vi "Save File DOE Find Individual Elements.vi"(11 "Input Array":string[](array[string])=["A", "a", "a", "B", "B", "c", "c", "C", "D", "E", "F", "F", "F", "G"]) -> (3 "Individual Elements":string[](array[string]))   [LabVIEW 2016, in "File Setup.lvlib"]
uses:
  File Setup.lvlib
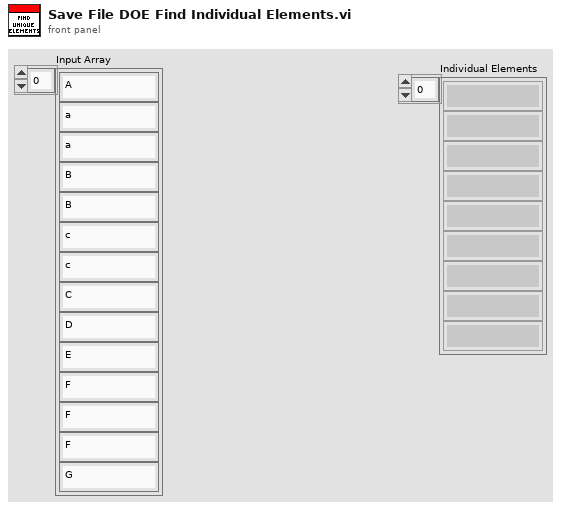
[diagram p1: front panel]
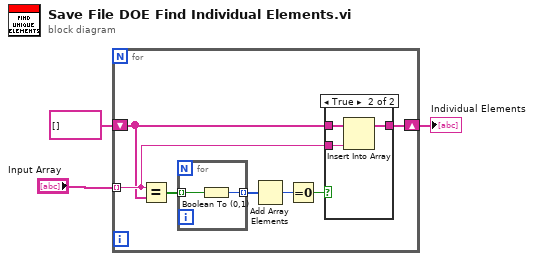
[diagram p0: block diagram]
diagram:
  n1 = for {
    tunnel: "Input Array" -> [w9] mode=indexing
    shift-right: [w10] -> w2
    shift-left: string[] [] -> [w8]
    n2 = Equal?(x=w9, y=w8) -> (x = y?=w7:bool[])
    n3 = for {
      tunnel: w7 -> [w12] mode=indexing
      tunnel: [w11] -> w6 mode=indexing
      n4 = Boolean To (0,1)(Boolean=w12) -> (0, 1=w11:i16)
    }
    n5 = Add Array Elements(numeric array=w6) -> (sum=w5:i16)
    n6 = Equal To 0?(x=w5) -> (x = 0?=w4:bool)
    n7 = case shown="True" w4 {
      tunnel: w9 -> [_ w16]
      tunnel: [w13 w15] -> w10
      tunnel: w8 -> [w13 w14]
      frame False {
      }
      frame True {
        n8 = Insert Into Array(array=w14, new element=w16) -> (w15:string[])  [unwired: 1 in]
      }
    }
  }
  "Individual Elements" <- w2
